vi "Main.vi"(8 "Error In":errorcluster, 11 "Simulate hardware?":bool) -> (0 "Error Out":errorcluster={"status"=FALSE, "code"=1073676418, "source"="VISA Close in Scope.lvlib:Main.vi->Top Level.vi"})   [LabVIEW 2017, in "Scope.lvlib"]
uses:
  Scope.lvlib
  Controls/Commands [enum].ctl
  Controls/Params.ctl
  Controls/Models.ctl
  Controls/TPC.ctl
  Controls/Channels.ctl
  Trigger/Controls/Params.ctl
  Trigger/Controls/Mode.ctl
  Trigger/Controls/Trigger channels.ctl
  Controls/Acquisition type.ctl
  Controls/Record length.ctl
  Controls/Data.ctl
  Controls/Channel data.ctl
  System Control/CTLs/Test params.ctl
  System Control/CTLs/Test Controls.ctl
  System Control/CTLs/Test indicators.ctl
  System Control/CTLs/Test Type.ctl
  File IO/Controls/Params.ctl
  Events/Controls/Action Refs [enum].ctl
  Events/Events.lvlib
  File IO/File IO.lvlib
  System Control/Main controller.lvlib
  Trigger/Trigger.lvlib
  UI/UI.lvlib
  Third Party Drivers/Tektronix DPO MSO 2000 4000 Series/Tektronix DPO MSO 2000 4000 Series.lvlib
panel:
  out "total time the scope will wait":dbl
  in  "wait multiplier":dbl=2500.0 format="%#_13g"
  in  "File IO parameters":T1={"Output Folder"=path "C:/Users/Abigail/Documents/Imperial Optical software/Optical Software Code Simplified/Output", "Error file"=path "Error Log.txt", "Config file"=path "Config.ini", "File prefix"="500 nm", "Waveform read"={"t0"=timestamp(0 s since 1904-01-01), "dt"=1.0, "Y"=[]}}
  out "TPC Final data":waveform(dbl)(graph)={"t0"=timestamp(3604925838.691944 s since 1904-01-01), "dt"=0.0004, "Y"=[2.0, 2.0, 2.0, 2.0, 2.0]}
  out "TAS Final data":waveform(dbl)(graph)={"t0"=timestamp(3604925838.691944 s since 1904-01-01), "dt"=0.0004, "Y"=[2.0, 2.0, 2.0, 2.0, 2.0]}
  out "TPC Averaged data":waveform(dbl)(graph)={"t0"=timestamp(3604925838.691944 s since 1904-01-01), "dt"=0.0004, "Y"=[2.0, 2.0, 2.0, 2.0, 2.0]}
  out "TPC Accumulated data":waveform(dbl)(graph)={"t0"=timestamp(3604925838.691944 s since 1904-01-01), "dt"=0.0004, "Y"=[]}
  out "TPC Live data":waveform(dbl)(graph)={"t0"=timestamp(3604925838.691944 s since 1904-01-01), "dt"=0.0004, "Y"=[1.0, 1.0, 1.0, 1.0, 1.0]}
  out "TAS Averaged data":waveform(dbl)(graph)={"t0"=timestamp(3604925838.691944 s since 1904-01-01), "dt"=0.0004, "Y"=[2.0, 2.0, 2.0, 2.0, 2.0]}
  out "TAS Accumulated data":waveform(dbl)(graph)={"t0"=timestamp(3604925838.691944 s since 1904-01-01), "dt"=0.0004, "Y"=[]}
  out "TAS Live data":waveform(dbl)(graph)={"t0"=timestamp(3604925838.691944 s since 1904-01-01), "dt"=0.0004, "Y"=[1.0, 1.0, 1.0, 1.0, 1.0]}
  out "Test":bool=TRUE
  out "Config out":T2={"Config"={"VISA Resource"="USB0::0x0699::0x039D::C010764::INSTR", "Model"=enum."DPO 2012B", "Timebase"=0.0004, "Timeout (ms)"=30000, "TAS"={"Vertical Range (V)"=0.2, "Vertical Offset (0.0 divs)"=0.4, "Bandwidth"=0, "Probe Attenuation (10.0)"=1.0, "Vertical Coupling"=1, "Impedance"=0, "Multiplication factor"=1.0, "Channel"=enum."Channel 1"}, "TPC"={"Vertical Range (V)"=0.2, "Vertical Offset (0.0 divs)"=0.0, "Bandwidth"=0, "Probe Attenuation (10.0)"=1.0, "Vertical Coupling"=1, "Impedance"=0, "Multiplication factor"=1.0, "Channel"=enum."B1"}, "Trigger"={"Mode"=enum."Laser (TAS)", "Source "=enum."Channel 2", "PIA"={"Test LEDs"=FALSE, "LED line"="", "LED off (s)"=1000.0, "LED on (s)"=1000.0}, "Threshold (V)"=0.8}}, "Indicators"={"Setup"={"Final number of points"=10000.0, "Pretrigger points"=1000.0, "Number of readouts"=5, "Model"={"Acquisition Type"=4, "Record length (points)"=1000, "Averages on scope"=4, "Average number of points"=100.0}}, "Timestamp of Data"=timestamp(0 s since 1904-01-01)}, "Data"={"TPC"={"Live data"={"t0"=timestamp(0 s since 1904-01-01), "dt"=0.0004, "Y"=array[10000 elements]}, "Averaged data"={"t0"=timestamp(0 s since 1904-01-01), "dt"=0.0004, "Y"=array[10000 elements]}, "Accumulated data"={"t0"=timestamp(0 s since 1904-01-01), "dt"=0.0004, "Y"=array[10000 elements]}, "Final data"={"t0"=timestamp(0 s since 1904-01-01), "dt"=1.0, "Y"=[]}}, "TAS"={"Live data"={"t0"=timestamp(0 s since 1904-01-01), "dt"=0.0004, "Y"=array[10000 elements]}, "Averaged data"={"t0"=timestamp(0 s since 1904-01-01), "dt"=0.0004, "Y"=array[10000 elements]}, "Accumulated data"={"t0"=timestamp(0 s since 1904-01-01), "dt"=0.0004, "Y"=array[10000 elements]}, "Final data"={"t0"=timestamp(0 s since 1904-01-01), "dt"=1.0, "Y"=[]}}, "Time arrays"={"Time array (decimated)"=[], "waveform"={"t0"=timestamp(0 s since 1904-01-01), "dt"=1.0, "Y"=[]}}}, "Test"={"Config"={"Amplification Factor"=0.0, "100% Reflectance Standard"=0.0, "Calculation Method"=enum."Reflectance", "Option to discard new data?"=FALSE, "Mode"=enum."Spectrum", "Number of Averages"=20, "B Test?"=FALSE}, "Indicators"={"DAQ Background Level (V)"=2.0, "A-Test Counter"=2, "B-Test Counter"=2, "Type"=enum."A-Test", "Scope Background Level (Amps)"=2.0, "TAS only?"=FALSE}}} {"Test"."Config"."Number of Averages" min=0; "Indicators"."Setup"."Model"."Record length (points)" items=["1000"=1, "10,000"=10, "100,000"=100, "1,000,000"=1000, "5,000,000"=5000, "10,000,000"=10000]; "Indicators"."Setup"."Model"."Acquisition Type" items=["Sample", "Peak Detect", "Hi Res", "Envelope", "Average"]; "Config"."Trigger"."Threshold (V)" format="%#_3f"; "Config"."TPC"."Impedance" items=["1M", "75", "50"]; "Config"."TPC"."Vertical Coupling" items=["AC", "DC", "Ground"]; "Config"."TPC"."Bandwidth" items=["FULL", "250 MHz", "150 MHz", "20 MHz"]; "Config"."TAS"."Impedance" items=["1M", "75", "50"]; "Config"."TAS"."Vertical Coupling" items=["AC", "DC", "Ground"]; "Config"."TAS"."Bandwidth" items=["FULL", "250 MHz", "150 MHz", "20 MHz"]; "Config"."Timebase" format="%^#_3e"}
  in  "Config":T2={"Config"={"VISA Resource"="USB0::0x0699::0x039D::C010764::INSTR", "Model"=enum."DPO 2012B", "Timebase"=0.0004, "Timeout (ms)"=30000, "TAS"={"Vertical Range (V)"=0.2, "Vertical Offset (0.0 divs)"=0.4, "Bandwidth"=0, "Probe Attenuation (10.0)"=1.0, "Vertical Coupling"=1, "Impedance"=0, "Multiplication factor"=1.0, "Channel"=enum."Channel 1"}, "TPC"={"Vertical Range (V)"=0.2, "Vertical Offset (0.0 divs)"=0.0, "Bandwidth"=0, "Probe Attenuation (10.0)"=1.0, "Vertical Coupling"=1, "Impedance"=0, "Multiplication factor"=1.0, "Channel"=enum."None"}, "Trigger"={"Mode"=enum."Laser (TAS)", "Source "=enum."Aux", "PIA"={"Test LEDs"=FALSE, "LED line"="", "LED off (s)"=1000.0, "LED on (s)"=1000.0}, "Threshold (V)"=0.8}}, "Indicators"={"Setup"={"Final number of points"=0.0, "Pretrigger points"=0.0, "Number of readouts"=0, "Model"={"Acquisition Type"=0, "Record length (points)"=10, "Averages on scope"=10, "Average number of points"=10000.0}}, "Timestamp of Data"=timestamp(0 s since 1904-01-01)}, "Data"={"TPC"={"Live data"={"t0"=timestamp(0 s since 1904-01-01), "dt"=1.0, "Y"=[]}, "Averaged data"={"t0"=timestamp(0 s since 1904-01-01), "dt"=1.0, "Y"=[]}, "Accumulated data"={"t0"=timestamp(0 s since 1904-01-01), "dt"=1.0, "Y"=[]}, "Final data"={"t0"=timestamp(0 s since 1904-01-01), "dt"=1.0, "Y"=[]}}, "TAS"={"Live data"={"t0"=timestamp(0 s since 1904-01-01), "dt"=1.0, "Y"=[]}, "Averaged data"={"t0"=timestamp(0 s since 1904-01-01), "dt"=1.0, "Y"=[]}, "Accumulated data"={"t0"=timestamp(0 s since 1904-01-01), "dt"=1.0, "Y"=[]}, "Final data"={"t0"=timestamp(0 s since 1904-01-01), "dt"=1.0, "Y"=[]}}, "Time arrays"={"Time array (decimated)"=[], "waveform"={"t0"=timestamp(0 s since 1904-01-01), "dt"=1.0, "Y"=[]}}}, "Test"={"Config"={"Amplification Factor"=2.0, "100% Reflectance Standard"=2.0, "Calculation Method"=enum."Reflectance", "Option to discard new data?"=FALSE, "Mode"=enum."Spectrum", "Number of Averages"=0, "B Test?"=FALSE}, "Indicators"={"DAQ Background Level (V)"=2.0, "A-Test Counter"=2, "B-Test Counter"=2, "Type"=enum."A-Test", "Scope Background Level (Amps)"=2.0, "TAS only?"=FALSE}}} {"Test"."Config"."Number of Averages" min=0; "Indicators"."Setup"."Model"."Record length (points)" items=["1000"=1, "10,000"=10, "100,000"=100, "1,000,000"=1000, "5,000,000"=5000, "10,000,000"=10000]; "Indicators"."Setup"."Model"."Acquisition Type" items=["Sample", "Peak Detect", "Hi Res", "Envelope", "Average"]; "Config"."Trigger"."Threshold (V)" format="%#_3f"; "Config"."TPC"."Impedance" items=["1M", "75", "50"]; "Config"."TPC"."Vertical Coupling" items=["AC", "DC", "Ground"]; "Config"."TPC"."Bandwidth" items=["FULL", "250 MHz", "150 MHz", "20 MHz"]; "Config"."TAS"."Impedance" items=["1M", "75", "50"]; "Config"."TAS"."Vertical Coupling" items=["AC", "DC", "Ground"]; "Config"."TAS"."Bandwidth" items=["FULL", "250 MHz", "150 MHz", "20 MHz"]; "Config"."Timebase" format="%^#_3e"}
  in  "Set state":T17=enum."Stop"
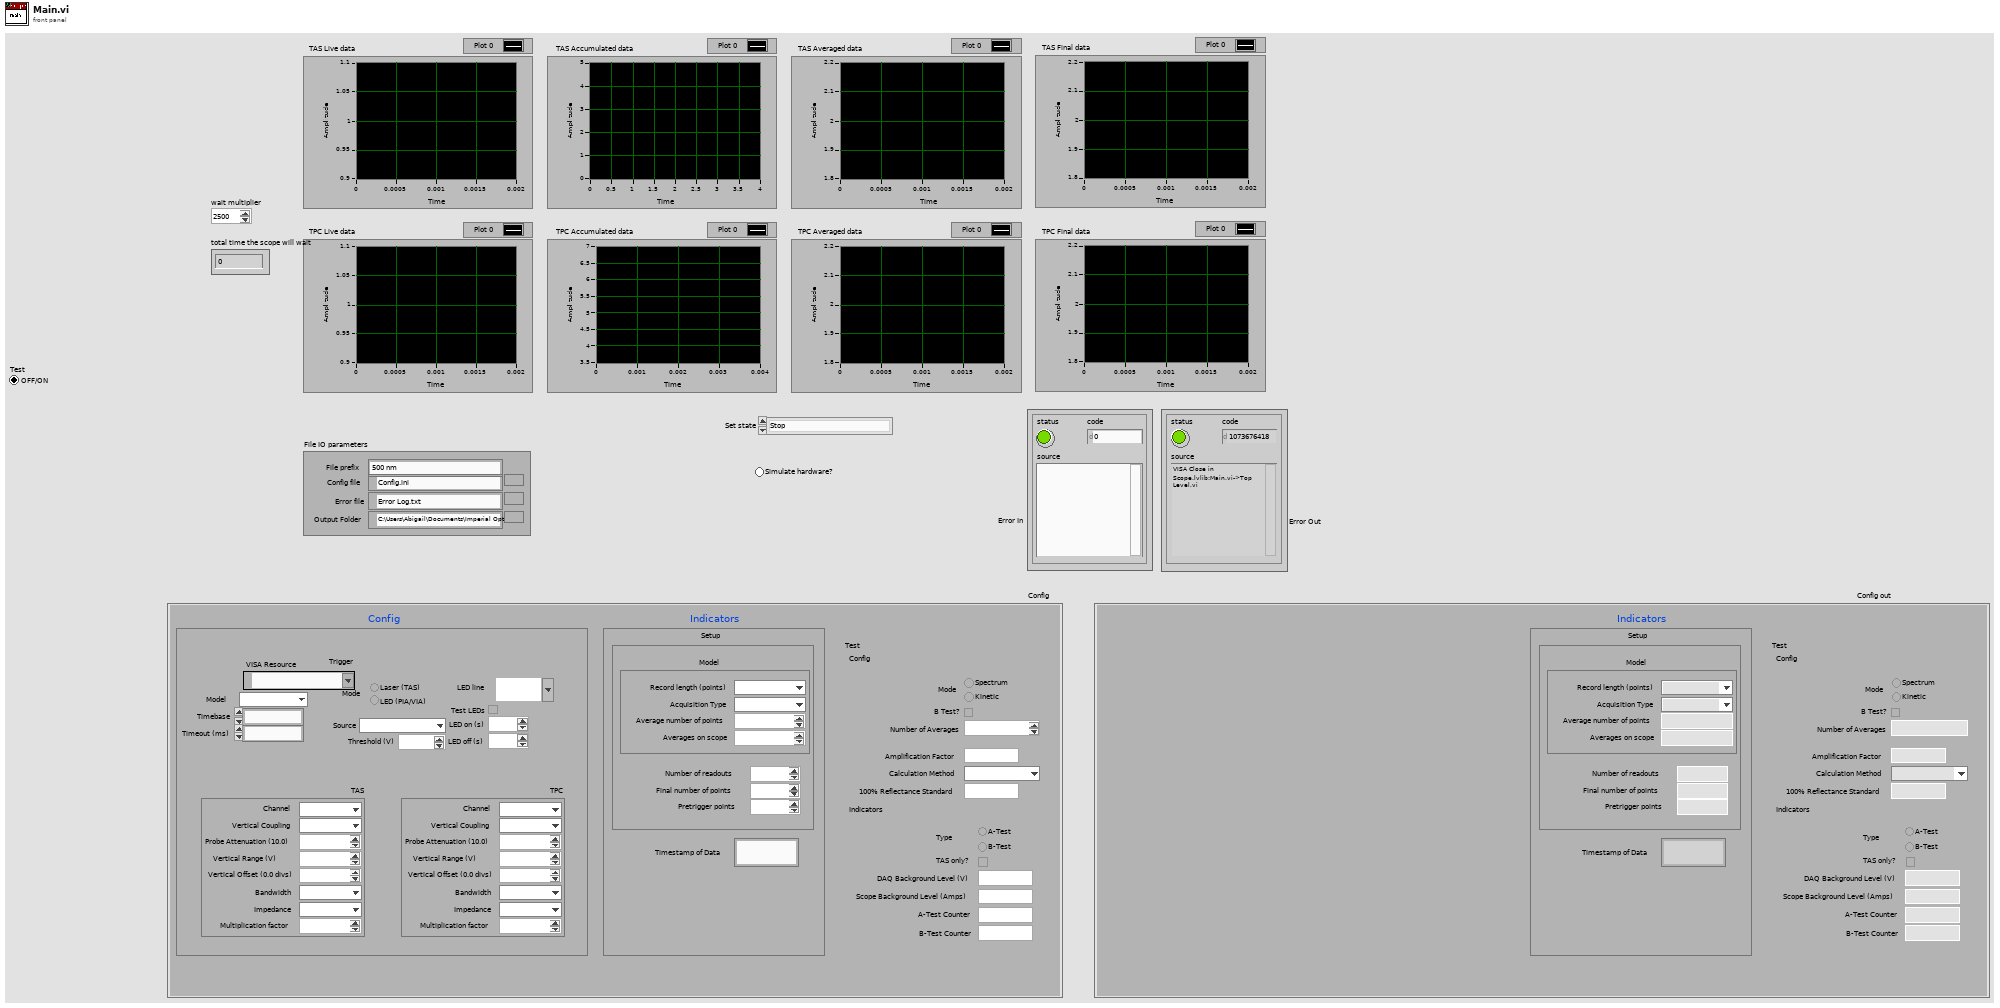
[diagram p1: front panel]
types:
  T1 = typedef "File IO.lvlib/Params.ctl" = cluster{"Output Folder":path, "Error file":path, "Config file":path, "File prefix":string, "Waveform read":waveform(dbl)}
  T2 = typedef "Scope.lvlib/Params.ctl" = cluster{"Config":cluster{"VISA Resource":refnum<visa-resource-name>, "Model":T3, "Timebase":dbl, "Timeout (ms)":u32, "TAS":T4, "TPC":T4, "Trigger":T6}, "Indicators":cluster{"Setup":cluster{"Final number of points":dbl, "Pretrigger points":dbl, "Number of readouts":i32, "Model":cluster{"Acquisition Type":T9, "Record length (points)":T10, "Averages on scope":i32, "Average number of points":dbl}}, "Timestamp of Data":timestamp}, "Data":T11, "Test":T13}
  T3 = typedef "Scope.lvlib/Models.ctl" = enum16{"DPO 3012", "DPO 2012B", "TDS 3012C"}
  T4 = typedef "Scope.lvlib/TPC.ctl" = cluster{"Vertical Range (V)":dbl, "Vertical Offset (0.0 divs)":dbl, "Bandwidth":i32, "Probe Attenuation (10.0)":dbl, "Vertical Coupling":u16, "Impedance":u16, "Multiplication factor":dbl, "Channel":T5}
  T5 = typedef "Scope.lvlib/Channels.ctl" = enum16{"Channel 1", "Channel 2", "Channel 3", "Channel 4", "Math", "Reference A", "Reference B", "Reference C", "Reference D", "B1", "B2", "None"}
  T6 = typedef "Scope.lvlib/Trigger.lvlib/Params.ctl" = cluster{"Mode":T7, "Source ":T8, "PIA":cluster{"Test LEDs":bool, "LED line":tag, "LED off (s)":dbl, "LED on (s)":dbl}, "Threshold (V)":dbl}
  T7 = typedef "Scope.lvlib/Trigger.lvlib/Mode.ctl" = enum32{"Laser (TAS)", "LED (PIA/VIA)"}
  T8 = typedef "Scope.lvlib/Trigger.lvlib/Trigger channels.ctl" = enum16{"Channel 1", "Channel 2", "Channel 3", "Channel 4", "AC Line", "Aux", "Digital Channel 0", "Digital Channel 1", "Digital Channel 2", "Digital Channel 3", "Digital Channel 4", "Digital Channel 5", "Digital Channel 6", "Digital Channel 7", "Digital Channel 8", "Digital Channel 9", "Digital Channel 10", "Digital Channel 11", "Digital Channel 12", "Digital Channel 13", "Digital Channel 14", "Digital Channel 15", "RF"}
  T9 = typedef "Scope.lvlib/Acquisition type.ctl" = u16
  T10 = typedef "Scope.lvlib/Record length.ctl" = u32
  T11 = typedef "Scope.lvlib/Data.ctl" = cluster{"TPC":T12, "TAS":T12, "Time arrays":cluster{"Time array (decimated)":dbl[], "waveform":waveform(dbl)}}
  T12 = typedef "Scope.lvlib/Channel data.ctl" = cluster{"Live data":waveform(dbl), "Averaged data":waveform(dbl), "Accumulated data":waveform(dbl), "Final data":waveform(dbl)}
  T13 = typedef "Main controller.lvlib/Test params.ctl" = cluster{"Config":T14, "Indicators":T15}
  T14 = typedef "Main controller.lvlib/Test Controls.ctl" = cluster{"Amplification Factor":dbl, "100% Reflectance Standard":dbl, "Calculation Method":enum16{"Reflectance", "Transmission", "Kubelka-Munk"}, "Option to discard new data?":bool, "Mode":enum32{"Spectrum", "Kinetic"}, "Number of Averages":i32, "B Test?":bool}
  T15 = typedef "Main controller.lvlib/Test indicators.ctl" = cluster{"DAQ Background Level (V)":dbl, "A-Test Counter":i32, "B-Test Counter":i32, "Type":T16, "Scope Background Level (Amps)":dbl, "TAS only?":bool}
  T16 = typedef "Main controller.lvlib/Test Type.ctl" = enum32{"A-Test", "B-Test"}
  T17 = typedef "Scope.lvlib/Commands [enum].ctl" = enum16{"Calculate parameters", "Start", "Stop", "Send data", "Start acquisition", "Get test data", "Accumulate test data", "Average test data", "Add background voltage", "Scale TPC", "Average Pre Trigger Data", "Write to file"}
  T18 = enum32{"Bad", "Idle", "Run top level", "Running"}
  T19 = typedef "Events.lvlib/Action Refs [enum].ctl" = enum16{"Init", "Ref", "Kill"}
  T20 = typedef "Events.lvlib/Refs [cluster].ctl" = cluster{"Exit":refnum<user-event>, "Controller":refnum<user-event>, "System Error":refnum<user-event>, "UI":refnum<user-event>, "Example Module":refnum<user-event>, "Shutter":refnum<user-event>, "Monochromator":refnum<user-event>, "DAQ":refnum<user-event>, "Scope":refnum<user-event>, "Processing":refnum<user-event>, "File IO":refnum<user-event>, "Colour wheel":refnum<user-event>}
  T21 = cluster{"Waveform Data":dbl[][], "Waveform name":string}
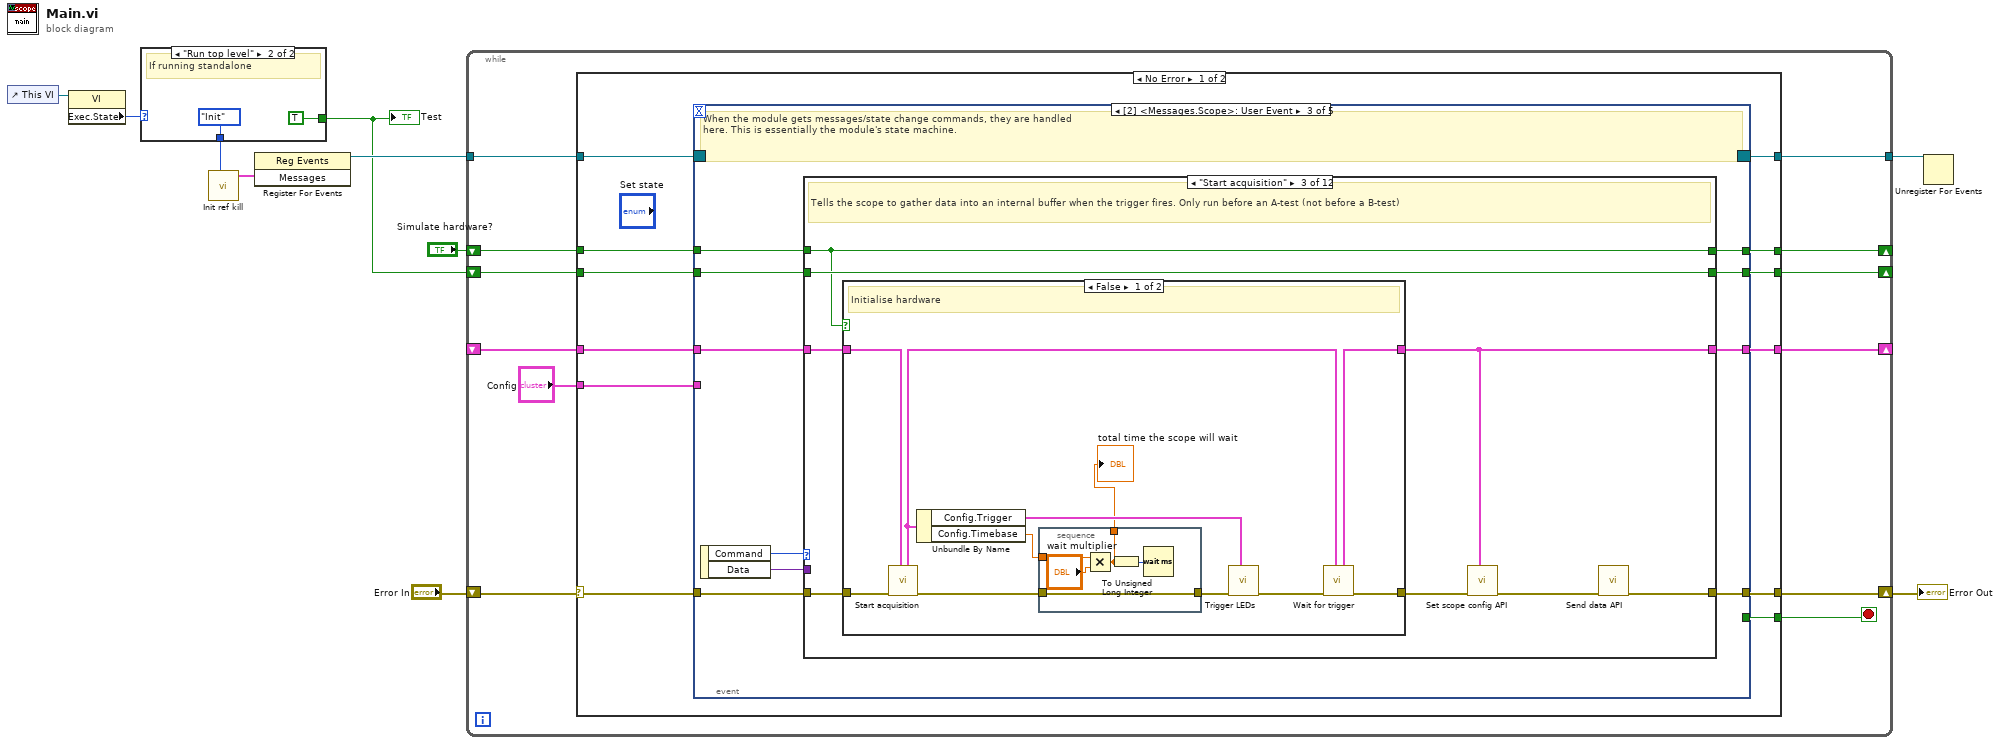
[diagram p0: block diagram]
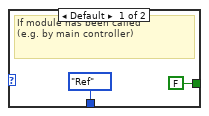
[diagram p2: hidden frame]
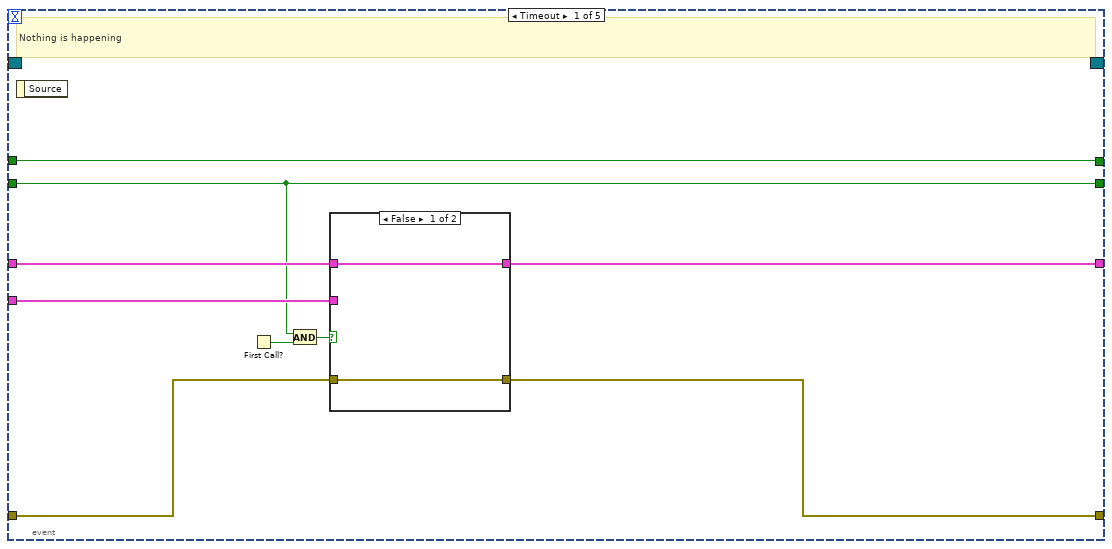
[diagram p3: hidden frame]
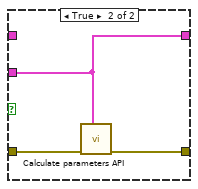
[diagram p4: hidden frame]
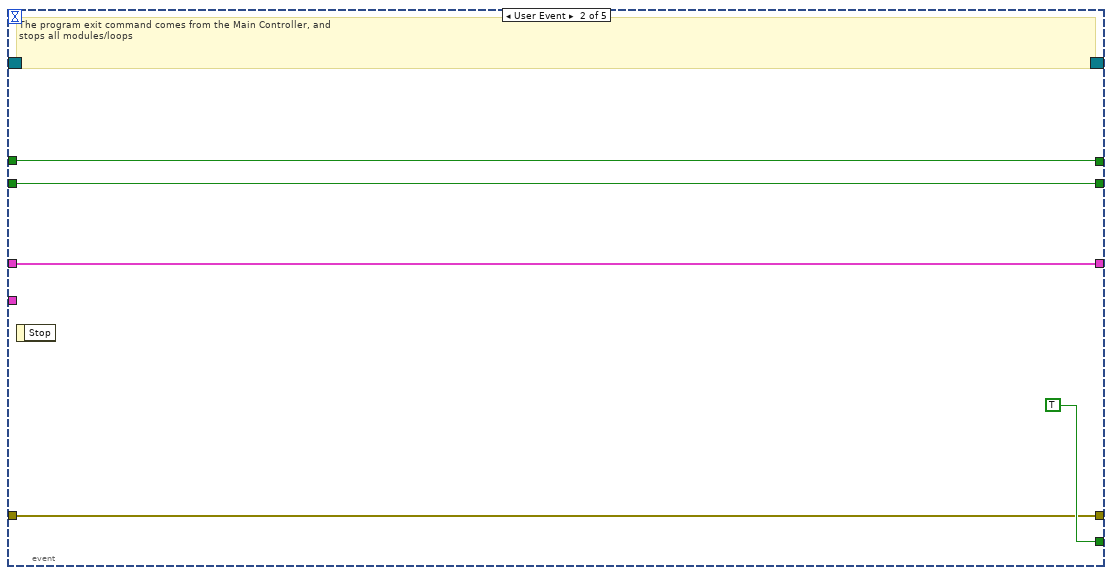
[diagram p5: hidden frame]
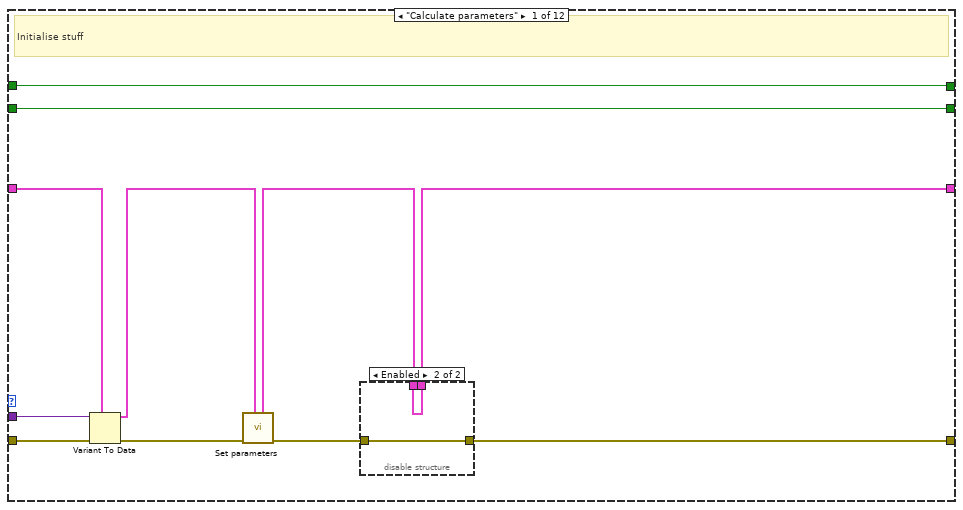
[diagram p6: hidden frame]
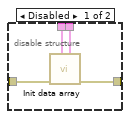
[diagram p7: hidden frame]
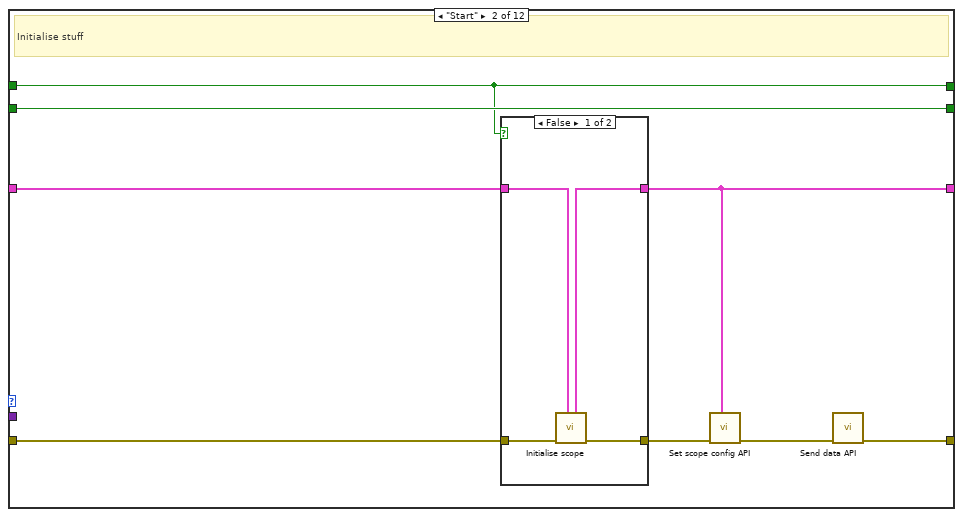
[diagram p8: hidden frame]
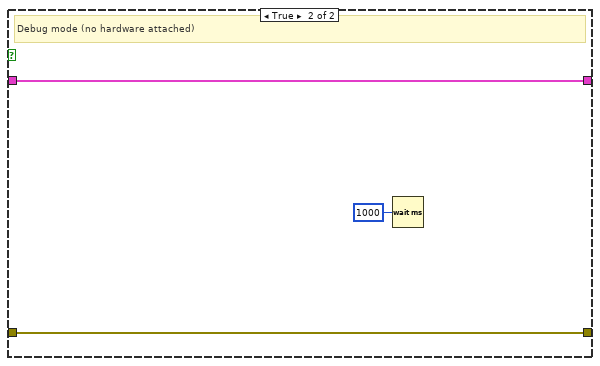
[diagram p10: hidden frame]
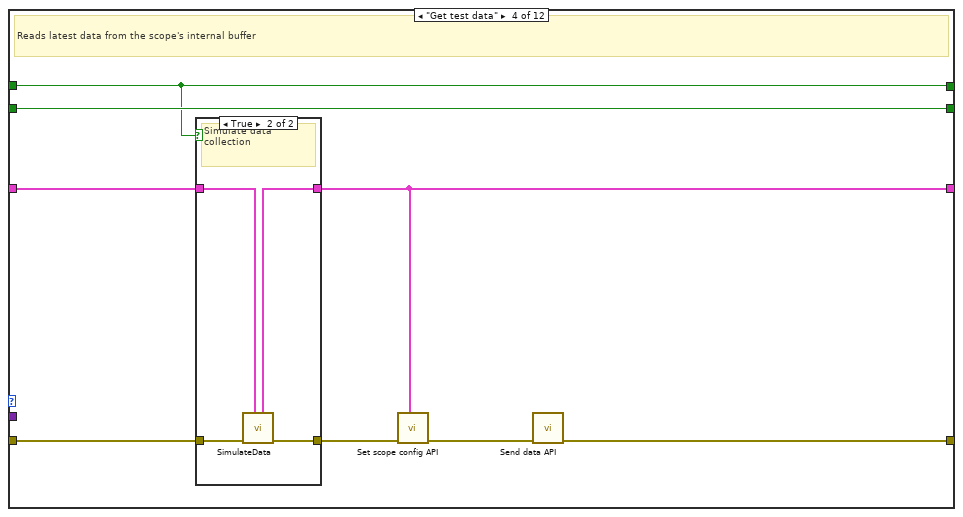
[diagram p11: hidden frame]
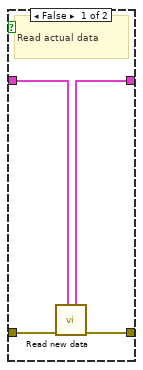
[diagram p12: hidden frame]
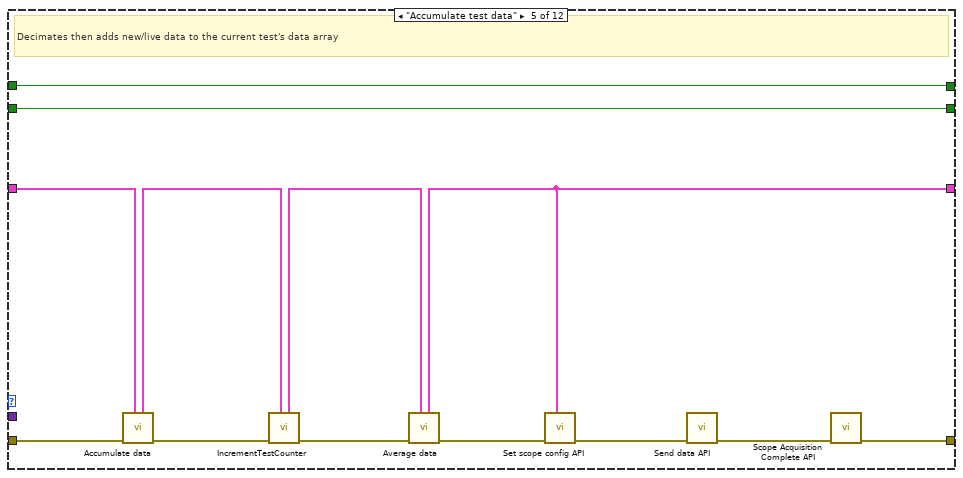
[diagram p13: hidden frame]
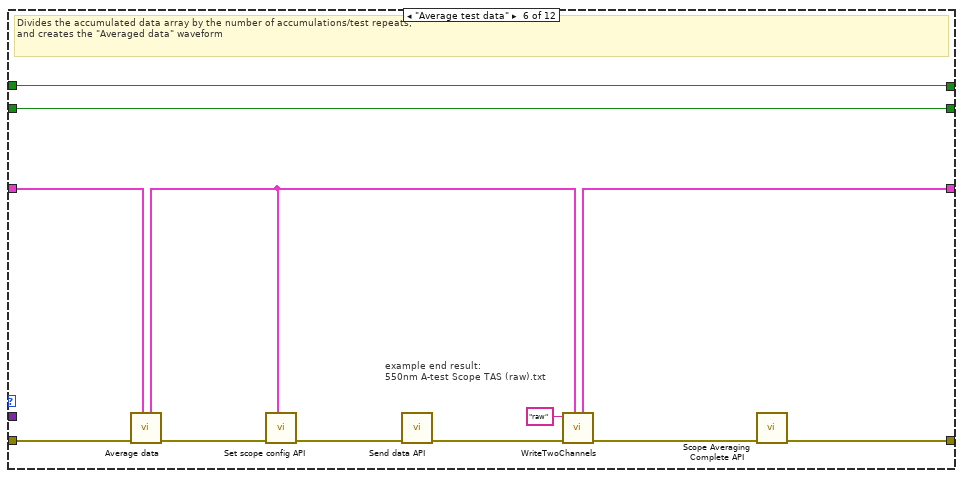
[diagram p14: hidden frame]
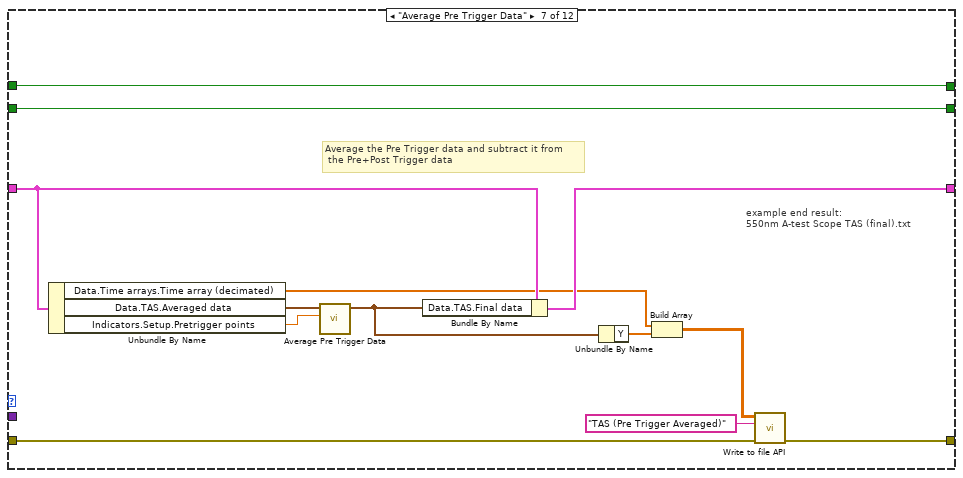
[diagram p15: hidden frame]
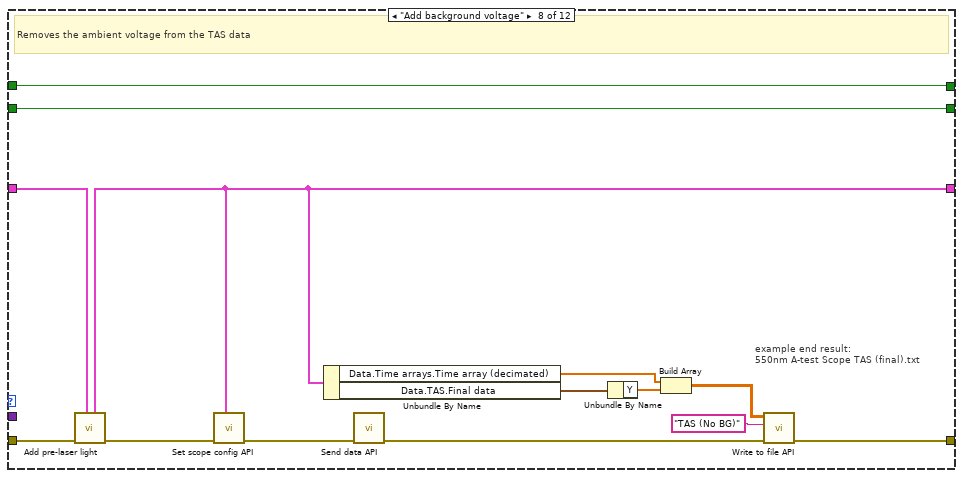
[diagram p16: hidden frame]
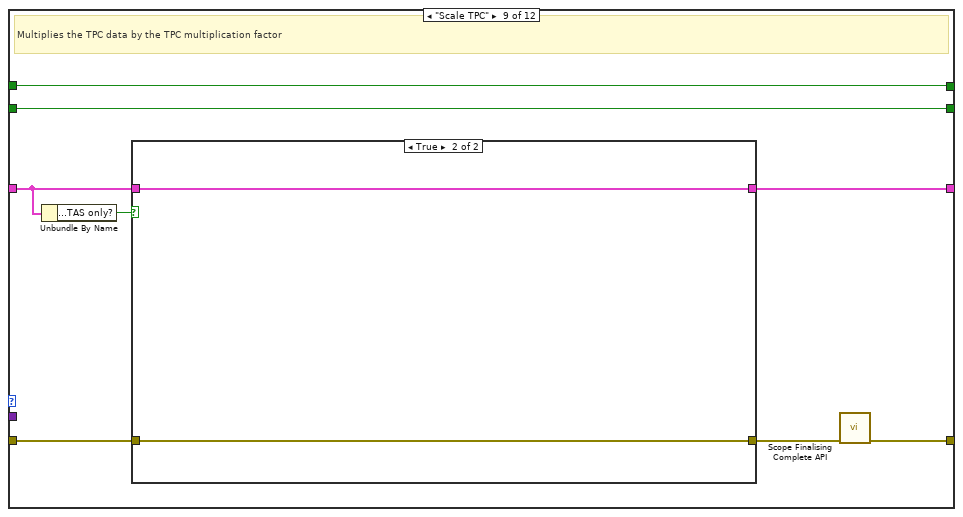
[diagram p17: hidden frame]
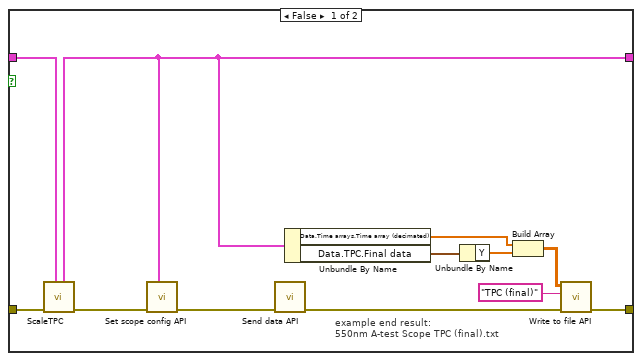
[diagram p18: hidden frame]
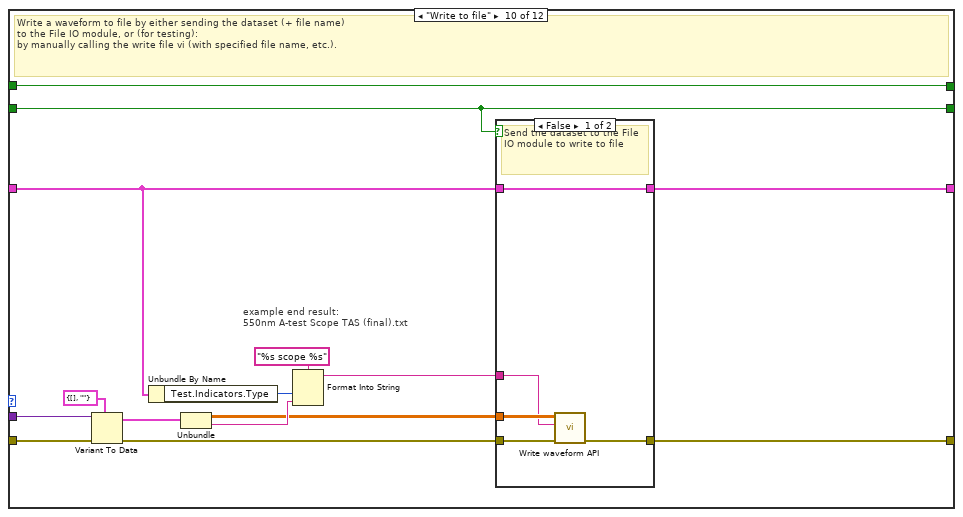
[diagram p19: hidden frame]
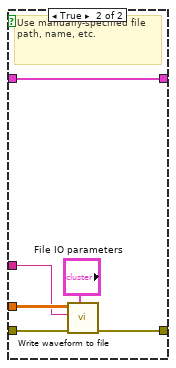
[diagram p20: hidden frame]
diagram:
  n1 = control-ref of="This VI"() -> (w5:refnum<vi>)
  n2 = property class="VI"(reference=w5) -> ("Exec.State"=w4:T18)  [unwired: 1 in, 2 out]
  n3 = case shown="\"Run top level\"" w4 {
    tunnel: [Action_Refs_[enum]."Ref" ("Action") Action_Refs_[enum]."Init" ("Action")] -> w3
    tunnel: [FALSE TRUE] -> w2
    frame Default {
      # "If module has been called\n(e.g. by main controller)"
    }
    frame "Run top level" {
      # "If running standalone"
    }
  }
  "Test" <- w2
  n4 = call "Init ref kill.vi"("Action"=w3) -> ("Messages"=w10:T20)  [unwired: 9 in, 1 out]
  n5 = register-events(w10) -> (reference out=w9:refnum<event-registration>)  [unwired: 2 in, 1 out]
  n6 = while {
    tunnel: w9 -> [w26]
    tunnel: [w24] -> w8
    shift-right: [w21] -> w6
    shift-left: "Error In" -> [w22]
    shift-right: [w20] -> _
    shift-left: _ -> [w23]
    shift-right: [w18] -> _
    shift-left: w2 -> [w19]
    shift-right: [w16] -> _
    shift-left: "Simulate hardware?" -> [w17]
    stop <- w25 stop-if-true
    n7 = case shown="No Error" w22 {
      selector: w22 -> [w32 w328]
      tunnel: w26 -> [w38 w326]
      tunnel: [w37 _] -> w25
      tunnel: [w36 w326] -> w24
      tunnel: w23 -> [w35 w327]
      tunnel: [w34 w327] -> w20
      tunnel: [w33 w329] -> w21
      tunnel: w19 -> [w31 w325]
      tunnel: [w30 w325] -> w18
      tunnel: w17 -> [w29 w324]
      tunnel: [w28 w324] -> w16
      tunnel: "Config" -> [w27 _]
      frame No Error {
        n8 = event shown="[2] <Messages.Scope>: User Event" {
          selector: w38 -> [_ _ _ _ _]
          dyn-events: [_ _ _ _ _] -> w36
          timeout: _ -> [_ _ _ _ _]
          tunnel: [_ TRUE _ _ _] -> w37
          tunnel: w32 -> [w44 w56 w65 w272 w280]
          tunnel: [w43 w56 w64 w271 w279] -> w33
          tunnel: w35 -> [w46 w55 w62 _ w281]
          tunnel: [w45 w55 w63 w273 w278] -> w34
          tunnel: w31 -> [w39 w54 w61 w275 w277]
          tunnel: [w39 w54 w60 w275 w277] -> w30
          tunnel: w29 -> [w47 w53 w59 w274 w276]
          tunnel: [w47 w53 w58 w274 w276] -> w28
          tunnel: w27 -> [w42 _ _ _ _]
          event Timeout {
            # "Nothing is happening"
            n9 = event-data() -> ()  [unwired: 1 in, 1 out]
            n10 = First Call?() -> (First Call?: T/F=w40:bool)
            n11 = And(x=w39, y=w40) -> (x .and. y?=w41:bool)
            n12 = case shown="False" w41 {
              tunnel: w46 -> [w49 _]
              tunnel: [w49 w50] -> w45
              tunnel: w44 -> [w48 w52]
              tunnel: [w48 w51] -> w43
              tunnel: w42 -> [_ w50]
              frame False {
              }
              frame True {
                n13 = call "Calculate parameters API.vi"("Scope"=w50, "Error In"=w52) -> ("Error Out"=w51:errorcluster)  [unwired: 9 in]
              }
            }
          }
          event User Event {
            # "The program exit command comes from the Main Controller, and \nstops all modules/loops"
            n14 = event-data() -> ()  [unwired: 1 in, 1 out]
          }
          event User Event {
            # "When the module gets messages/state change commands, they are handled \nhere. This is essentially the module's state machine."
            n15 = event-data() -> ("Command"=w67:T17, "Data"=w66:variant)  [unwired: 1 in]
            n16 = case shown="\"Start acquisition\"" w67 {
              tunnel: w66 -> [w77 _ _ _ _ _ _ _ _ w228 _ _]
              tunnel: w65 -> [w78 w89 w106 w132 w154 w166 w170 w192 w200 w229 w244 w265]
              tunnel: [w68 w88 w102 w129 w149 w158 w169 w187 w196 w219 w242 w260] -> w64
              tunnel: w62 -> [w76 w90 w103 w133 w152 w165 w176 w193 w195 w225 w243 w262]
              tunnel: [w69 w85 w99 w126 w147 w161 w175 w180 w199 w230 w243 w259] -> w63
              tunnel: w61 -> [w71 w92 w105 w131 w153 w164 w179 w191 w201 w227 w246 w266]
              tunnel: [w71 w92 w105 w131 w153 w164 w179 w191 w201 w227 w246 w266] -> w60
              tunnel: [w70 w91 w104 w130 w151 w160 w178 w188 w198 w220 w245 w263] -> w58
              tunnel: w59 -> [w70 w91 w104 w130 w151 w160 w178 w188 w198 w220 w245 w263]
              frame "Calculate parameters" {
                # "Initialise stuff"
                n17 = Variant To Data(error in=w78, type=w76, Variant=w77) -> (data=w75:T2, error out=w74:errorcluster)
                n18 = call "Set parameters.vi"("Scope"=w75, "error in"=w74) -> ("error out"=w72:errorcluster, "Scope out"=w73:T2)  [unwired: 8 in]
                n19 = disable-structure shown="Enabled" {
                  disable-tunnel: w73 -> [w82 w83]
                  disable-tunnel: w72 -> [w81 w84]
                  disable-tunnel: [w80 w83] -> w69
                  disable-tunnel: [w79 w84] -> w68
                  frame Disabled {
                    n20 = call "Init data array.vi"("Scope in"=w82, "error in (no error)"=w81) -> ("error out"=w79:errorcluster, "Scope out"=w80:T2)  [unwired: 8 in]
                  }
                  frame Enabled {
                  }
                }
              }
              frame "Start" {
                # "Initialise stuff"
                n21 = case shown="False" w91 {
                  tunnel: [w95 w97] -> w85
                  tunnel: [w96 w98] -> w87
                  tunnel: w90 -> [w94 w97]
                  tunnel: w89 -> [w93 w98]
                  frame False {
                    n22 = call "Initialise scope.vi"("Config"=w94, "error in (no error)"=w93) -> ("error out"=w96:errorcluster, "Scope out"=w95:T2)  [unwired: 8 in]
                  }
                  frame True {
                    # "In debug mode"
                  }
                }
                n23 = call "Set scope config API.vi"("Scope"=w85, "Error In"=w87) -> ("Error Out"=w86:errorcluster)  [unwired: 9 in]
                n24 = call "Send data API.vi"("Error In"=w86) -> ("Error Out"=w88:errorcluster)  [unwired: 10 in]
              }
              frame "Start acquisition" {
                # "Tells the scope to gather data into an internal buffer when the trigger fires. Only run before an A-test (not before a B-test)"
                n25 = case shown="False" w104 {
                  tunnel: w103 -> [w114 w124]
                  tunnel: [w113 w124] -> w99
                  tunnel: [w112 w123] -> w101
                  tunnel: w106 -> [w111 w123]
                  frame False {
                    # "Initialise hardware"
                    n26 = call "Start acquisition.vi"("Scope in"=w114, "error in (no error)"=w111) -> ("error out"=w110:errorcluster, "Scope out"=w116:T2)  [unwired: 8 in]
                    n27 = Unbundle By Name(w116) -> ("Config.Trigger"=w117:T6, "Config.Timebase"=w108:dbl)
                    n28 = stacked-sequence {
                      tunnel: w110 -> [w122]
                      tunnel: [w122] -> w109
                      tunnel: w108 -> [w120]
                      tunnel: [w118] -> w107
                      frame #0 {
                        n29 = Multiply(x=w120, y="wait multiplier") -> (x*y=w118:dbl)
                        n30 = To Unsigned Long Integer(number=w118) -> (unsigned 32bit integer=w119:u32)
                        n31 = Wait (ms)(milliseconds to wait=w119) -> ()  [unwired: 1 out]
                      }
                    }
                    "total time the scope will wait" <- w107
                    n32 = call "Trigger LEDs.vi"("Trigger"=w117, "error in (no error)"=w109) -> ("error out"=w115:errorcluster)  [unwired: 9 in]
                    n33 = call "Wait for trigger.vi"("Scope"=w116, "error in (no error)"=w115) -> ("error out"=w112:errorcluster, "Scope out"=w113:T2)  [unwired: 8 in]
                  }
                  frame True {
                    # "Debug mode (no hardware attached)"
                    n34 = Wait (ms)(milliseconds to wait=u32 1000) -> ()  [unwired: 1 out]
                  }
                }
                n35 = call "Set scope config API.vi"("Scope"=w99, "Error In"=w101) -> ("Error Out"=w100:errorcluster)  [unwired: 9 in]
                n36 = call "Send data API.vi"("Error In"=w100) -> ("Error Out"=w102:errorcluster)  [unwired: 10 in]
              }
              frame "Get test data" {
                # "Reads latest data from the scope's internal buffer"
                n37 = case shown="True" w130 {
                  tunnel: [w136 w140] -> w127
                  tunnel: w132 -> [w137 w141]
                  tunnel: w133 -> [w135 w139]
                  tunnel: [w134 w138] -> w126
                  frame False {
                    # "Read actual data"
                    n38 = call "Read new data.vi"("Scope"=w135, "error in (no error)"=w137) -> ("error out"=w136:errorcluster, "Scope out"=w134:T2)  [unwired: 7 in, 1 out]
                  }
                  frame True {
                    # "Simulate data collection"
                    n39 = call "SimulateData.vi"("Scope"=w139, "error in (no error)"=w141) -> ("error out"=w140:errorcluster, "Scope out"=w138:T2)  [unwired: 8 in]
                  }
                }
                n40 = call "Set scope config API.vi"("Scope"=w126, "Error In"=w127) -> ("Error Out"=w128:errorcluster)  [unwired: 9 in]
                n41 = call "Send data API.vi"("Error In"=w128) -> ("Error Out"=w129:errorcluster)  [unwired: 10 in]
              }
              frame "Accumulate test data" {
                # "Decimates then adds new/live data to the current test's data array"
                n42 = call "Accumulate data.vi"("Scope"=w152, "error in"=w154) -> ("error out"=w144:errorcluster, "Scope out"=w143:T2)  [unwired: 8 in]
                n43 = call "IncrementTestCounter.vi"("Scope"=w143, "error in"=w144) -> ("error out"=w145:errorcluster, "Scope out"=w142:T2)  [unwired: 8 in]
                n44 = call "Average data.vi"("Scope"=w142, "error in"=w145) -> ("error out"=w146:errorcluster, "Scope out"=w147:T2)  [unwired: 8 in]
                n45 = call "Set scope config API.vi"("Scope"=w147, "Error In"=w146) -> ("Error Out"=w148:errorcluster)  [unwired: 9 in]
                n46 = call "Send data API.vi"("Error In"=w148) -> ("Error Out"=w150:errorcluster)  [unwired: 10 in]
                n47 = call "Scope Acquisition Complete API.vi"("Error In"=w150) -> ("Error Out"=w149:errorcluster)  [unwired: 10 in]
              }
              frame "Average test data" {
                # "example end result:\n550nm A-test Scope TAS (raw).txt"
                # "Divides the accumulated data array by the number of accumulations/test repeats, \nand creates the \"Averaged data\" waveform"
                n48 = call "Average data.vi"("Scope"=w165, "error in"=w166) -> ("error out"=w157:errorcluster, "Scope out"=w155:T2)  [unwired: 8 in]
                n49 = call "Set scope config API.vi"("Scope"=w155, "Error In"=w157) -> ("Error Out"=w156:errorcluster)  [unwired: 9 in]
                n50 = call "Send data API.vi"("Error In"=w156) -> ("Error Out"=w162:errorcluster)  [unwired: 10 in]
                n51 = call "WriteTwoChannels.vi"("Scope in"=w155, "error in (no error)"=w162, "Waveform name"="raw") -> ("error out"=w159:errorcluster, "Scope out"=w161:T2)  [unwired: 7 in]
                n52 = call "Scope Averaging Complete API.vi"("Error In"=w159) -> ("Error Out"=w158:errorcluster)  [unwired: 10 in]
              }
              frame "Average Pre Trigger Data" {
                # "Average the Pre Trigger data and subtract it from\n the Pre+Post Trigger data"
                # "example end result:\n550nm A-test Scope TAS (final).txt"
                n53 = Unbundle By Name(w176) -> ("Data.Time arrays.Time array (decimated)"=w168:dbl[], "Data.TAS.Averaged data"=w174:waveform(dbl), "Indicators.Setup.Pretrigger points"=w177:dbl)
                n54 = call "Average Pre Trigger Data.vi"("Pretrigger points"=w177, "Averaged data in"=w174) -> ("Averaged data out"=w167:waveform(dbl))  [unwired: 9 in]
                n55 = Bundle By Name(cluster=w176, "Data.TAS.Final data"=w167) -> (w175:T2)
                n56 = Unbundle By Name(w167) -> ("Y"=w172:dbl[])
                n57 = Build Array(w168, w172) -> (w173:dbl[][])
                n58 = call "Write to file API.vi"("Error In"=w170, "Waveform name"="TAS (Pre Trigger Averaged)", "Waveform Data"=w173) -> ("Error Out"=w169:errorcluster)  [unwired: 8 in]
              }
              frame "Add background voltage" {
                # "example end result:\n550nm A-test Scope TAS (final).txt"
                # "Removes the ambient voltage from the TAS data"
                n59 = call "Add pre-laser light.vi"("Scope"=w193, "error in"=w192) -> ("error out"=w182:errorcluster, "Scope out"=w180:T2)  [unwired: 8 in]
                n60 = call "Set scope config API.vi"("Scope"=w180, "Error In"=w182) -> ("Error Out"=w181:errorcluster)  [unwired: 9 in]
                n61 = Unbundle By Name(w180) -> ("Data.Time arrays.Time array (decimated)"=w183:dbl[], "Data.TAS.Final data"=w185:waveform(dbl))
                n62 = call "Send data API.vi"("Error In"=w181) -> ("Error Out"=w190:errorcluster)  [unwired: 10 in]
                n63 = Unbundle By Name(w185) -> ("Y"=w186:dbl[])
                n64 = Build Array(w183, w186) -> (w184:dbl[][])
                n65 = call "Write to file API.vi"("Error In"=w190, "Waveform name"="TAS (No BG)", "Waveform Data"=w184) -> ("Error Out"=w187:errorcluster)  [unwired: 8 in]
              }
              frame "Scale TPC" {
                # "Multiplies the TPC data by the TPC multiplication factor"
                n66 = Unbundle By Name(w195) -> ("Test.Indicators.TAS only?"=w194:bool)
                n67 = case shown="True" w194 {
                  tunnel: w200 -> [w213 w214]
                  tunnel: [w202 w215] -> w199
                  tunnel: [w210 w214] -> w197
                  tunnel: w195 -> [w206 w215]
                  frame False {
                    # "example end result:\n550nm A-test Scope TPC (final).txt"
                    n68 = call "ScaleTPC.vi"("Scope in"=w206, "Error In"=w213) -> ("Error Out"=w204:errorcluster, "Scope out"=w202:T2)  [unwired: 8 in]
                    n69 = call "Set scope config API.vi"("Scope"=w202, "Error In"=w204) -> ("Error Out"=w203:errorcluster)  [unwired: 9 in]
                    n70 = call "Send data API.vi"("Error In"=w203) -> ("Error Out"=w211:errorcluster)  [unwired: 10 in]
                    n71 = Unbundle By Name(w202) -> ("Data.Time arrays.Time array (decimated)"=w205:dbl[], "Data.TPC.Final data"=w209:waveform(dbl))
                    n72 = Unbundle By Name(w209) -> ("Y"=w208:dbl[])
                    n73 = Build Array(w205, w208) -> (w207:dbl[][])
                    n74 = call "Write to file API.vi"("Error In"=w211, "Waveform name"="TPC (final)", "Waveform Data"=w207) -> ("Error Out"=w210:errorcluster)  [unwired: 8 in]
                  }
                  frame True {
                  }
                }
                n75 = call "Scope Finalising Complete API.vi"("Error In"=w197) -> ("Error Out"=w196:errorcluster)  [unwired: 10 in]
              }
              frame "Write to file" {
                # "example end result:\n550nm A-test Scope TAS (final).txt"
                # "Write a waveform to file by either sending the dataset (+ file name) \nto the File IO module, or (for testing):\nby manually calling the write file vi (with specified file name, etc.)."
                n76 = Variant To Data(error in=w229, type=T21 {"Waveform Data"=[], "Waveform name"=""} ("output cluster"), Variant=w228) -> (data=w223:T21, error out=w226:errorcluster)
                n77 = Unbundle By Name(w225) -> ("Test.Indicators.Type"=w218:T16)
                n78 = Unbundle(w223) -> ("Waveform Data"=w217:dbl[][], "Waveform name"=w222:string)
                n79 = Format Into String(format string="%s scope %s", w218, w222) -> (resulting string=w221:string)  [unwired: 2 in, 1 out]
                n80 = case shown="False" w227 {
                  tunnel: [w235 w241] -> w219
                  tunnel: w225 -> [w234 w240]
                  tunnel: [w234 w240] -> w230
                  tunnel: w217 -> [w233 w239]
                  tunnel: w226 -> [w232 w238]
                  tunnel: w221 -> [w231 w237]
                  frame False {
                    # "Send the dataset to the File IO module to write to file"
                    n81 = call "Write waveform API.vi"("Error In"=w232, "Waveform name"=w231, "Waveform Data"=w233) -> ("Error Out"=w235:errorcluster)  [unwired: 8 in]
                  }
                  frame True {
                    # "Use manually-specified file path, name, etc."
                    n82 = call "Write waveform to file.vi"("File IO parameters"="File IO parameters", "error in"=w238, "Dataset name"=w237, "Data"=w239) -> ("error out"=w241:errorcluster)  [unwired: 7 in]
                  }
                }
              }
              frame "Send data" {
                # "Send a message to the UI module to update the display \nwith the new data/config, and update the master controller\nwith the module config."
                n83 = Unbundle By Name(w243) -> ("Data.TAS"=w252:T12)
                n84 = Unbundle By Name(w243) -> ("Data.TPC"=w251:T12)
                n85 = Unbundle By Name(w252) -> ("Live data"=→"TAS Live data":waveform(dbl), "Accumulated data"=→"TAS Accumulated data":waveform(dbl), "Averaged data"=→"TAS Averaged data":waveform(dbl), "Final data"=→"TAS Final data":waveform(dbl))
                n86 = Unbundle By Name(w251) -> ("Live data"=→"TPC Live data":waveform(dbl), "Accumulated data"=→"TPC Accumulated data":waveform(dbl), "Averaged data"=→"TPC Averaged data":waveform(dbl), "Final data"=→"TPC Final data":waveform(dbl))
                n87 = call "Set scope data API.vi"("Scope"=w243, "Error In"=w244) -> ("Error Out"=w242:errorcluster)  [unwired: 9 in]
                "Config out" <- w243
              }
              frame "Stop" {
                # "Close stuff"
                n88 = Unbundle By Name(w262) -> ("Config.VISA Resource"=w264:refnum<visa-resource-name>)  [unwired: 2 out]
                n89 = case shown="True" w263 {
                  tunnel: [w269 w270] -> w261
                  tunnel: w265 -> [w268 w270]
                  tunnel: w264 -> [w267 _]
                  frame False {
                    n90 = call "Close.vi"("error in (no error)"=w268, "VISA resource name"=w267) -> ("error out"=w269:errorcluster)  [unwired: 9 in]
                  }
                  frame True {
                  }
                }
                n91 = Bundle By Name(cluster=w262, "Data"=T11 {"TPC"={"Live data"={"t0"=timestamp(0 s since 1904-01-01), "dt"=1.0, "Y"=[]}, "Averaged data"={"t0"=timestamp(0 s since 1904-01-01), "dt"=1.0, "Y"=[]}, "Accumulated data"={"t0"=timestamp(0 s since 1904-01-01), "dt"=1.0, "Y"=[]}, "Final data"={"t0"=timestamp(0 s since 1904-01-01), "dt"=1.0, "Y"=[]}}, "TAS"={"Live data"={"t0"=timestamp(0 s since 1904-01-01), "dt"=1.0, "Y"=[]}, "Averaged data"={"t0"=timestamp(0 s since 1904-01-01), "dt"=1.0, "Y"=[]}, "Accumulated data"={"t0"=timestamp(0 s since 1904-01-01), "dt"=1.0, "Y"=[]}, "Final data"={"t0"=timestamp(0 s since 1904-01-01), "dt"=1.0, "Y"=[]}}, "Time arrays"={"Time array (decimated)"=[], "waveform"={"t0"=timestamp(0 s since 1904-01-01), "dt"=1.0, "Y"=[]}}}, "Test.Indicators"=T15 {"DAQ Background Level (V)"=0.0, "A-Test Counter"=0, "B-Test Counter"=0, "Type"=enum."A-Test", "Scope Background Level (Amps)"=0.0, "TAS only?"=FALSE}) -> (w259:T2)
                n92 = call "Set scope config API.vi"("Scope"=w259, "Error In"=w261) -> ("Error Out"=w260:errorcluster)  [unwired: 9 in]
              }
            }
          }
          event Value Change {
            n93 = event-data() -> ("NewVal"=w273:T2)  [unwired: 1 in]
            n94 = call "Calculate parameters API.vi"("Scope"=w273, "Error In"=w272) -> ("Error Out"=w271:errorcluster)  [unwired: 9 in]
          }
          event Value Change {
            # "By changing the \"Set state\" dropdown, you can manually put the scope \nmodule/state machine into particular states (for testing)"
            n95 = event-data() -> ("NewVal"=w282:T17)  [unwired: 1 in]
            n96 = case shown="\"Average Pre Trigger Data\"" w282 {
              tunnel: w281 -> [w283 w286 w291 w292 w296 w301 w304 w307 w309 w312 w315 w318]
              tunnel: [w283 w286 w291 w292 w296 w301 w304 w307 w309 w312 w315 w318] -> w278
              tunnel: [w284 w287 w289 w295 w297 w299 w302 w305 w308 w310 w313 w323] -> w279
              tunnel: w280 -> [w285 w288 w290 w294 w298 w300 w303 w306 w308 w311 w314 w322]
              frame "Calculate parameters" {
                n97 = call "Calculate parameters API.vi"("Scope"=w283, "Error In"=w285) -> ("Error Out"=w284:errorcluster)  [unwired: 9 in]
              }
              frame "Start" {
                n98 = call "Start API.vi"("Error In"=w288) -> ("Error Out"=w287:errorcluster)  [unwired: 10 in]
              }
              frame "Stop" {
                n99 = call "Stop API.vi"("Error In"=w290) -> ("Error Out"=w289:errorcluster)  [unwired: 10 in]
              }
              frame "Send data" {
                n100 = call "Set scope config API.vi"("Scope"=w292, "Error In"=w294) -> ("Error Out"=w293:errorcluster)  [unwired: 9 in]
                n101 = call "Send data API.vi"("Error In"=w293) -> ("Error Out"=w295:errorcluster)  [unwired: 10 in]
              }
              frame "Start acquisition" {
                n102 = call "Start acquisition API.vi"("Error In"=w298) -> ("Error Out"=w297:errorcluster)  [unwired: 10 in]
              }
              frame "Get test data" {
                n103 = call "Get test data API.vi"("Error In"=w300) -> ("Error Out"=w299:errorcluster)  [unwired: 10 in]
              }
              frame "Accumulate test data" {
                n104 = call "Accumulate data API.vi"("Error In"=w303) -> ("Error Out"=w302:errorcluster)  [unwired: 10 in]
              }
              frame "Average test data" {
                n105 = call "Average data API.vi"("Error In"=w306) -> ("Error Out"=w305:errorcluster)  [unwired: 10 in]
              }
              frame "Average Pre Trigger Data" {
              }
              frame "Add background voltage" {
                n106 = call "Add background voltage API.vi"("Error In"=w311) -> ("Error Out"=w310:errorcluster)  [unwired: 10 in]
              }
              frame "Scale TPC" {
                n107 = call "Scale TPC API.vi"("Error In"=w314) -> ("Error Out"=w313:errorcluster)  [unwired: 10 in]
              }
              frame "Write to file" {
                n108 = Unbundle By Name(w318) -> ("Data.Time arrays.Time array (decimated)"=w316:dbl[], "Data.TPC.Final data"=w320:waveform(dbl))
                n109 = Unbundle By Name(w320) -> ("Y"=w319:dbl[])
                n110 = Build Array(w316, w319) -> (w317:dbl[][])
                n111 = call "Write to file API.vi"("Error In"=w322, "Waveform name"="CH1 (final)", "Waveform Data"=w317) -> ("Error Out"=w323:errorcluster)  [unwired: 8 in]
              }
            }
          }
        }
      }
      frame Error {
        n112 = local read "Test"() -> (w330:bool)
        n113 = case shown="False" w330 {
          tunnel: [w332 _] -> w329
          tunnel: w328 -> [w331 w337]
          frame False {
            n114 = case shown="Error" w331 {
              selector: w331 -> [w333 w335]
              tunnel: [w333 w336] -> w332
              frame No Error {
              }
              frame Error {
                n115 = call "Send Error API.vi"("Error Cluster"=w335) -> ("Error Out"=w334:errorcluster)  [unwired: 10 in]
                n116 = call "Log error API.vi"("Error In"=w334) -> ("Error Out"=w336:errorcluster)  [unwired: 10 in]
              }
            }
          }
          frame True {
            n117 = call <vilib>:"Simple Error Handler.vi"("error in (no error)"=w337) -> ()  [unwired: 4 in, 5 out]
          }
        }
      }
    }
  }
  "Error Out" <- w6
  n118 = Unregister For Events(event registration refnum=w8) -> ()  [unwired: 1 in, 1 out]
